vi "Get Plugin Name.vi"(8 "error in (no error)":errorcluster, 11 "Python Protocol in":refnum<class "Python Protocol.lvclass">) -> (0 "error out":errorcluster, 2 "String":string, 3 "Python Protocol out":refnum<class "Python Protocol.lvclass">)   [LabVIEW 2013, in "Python Protocol.lvlib" / "Python Protocol.lvclass"]
uses:
  Python Protocol.lvclass
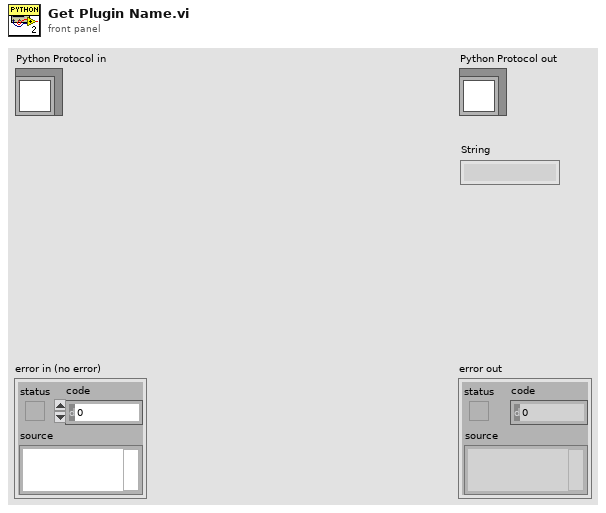
[diagram p1: front panel]
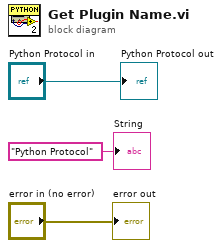
[diagram p0: block diagram]
diagram:
  "error out" <- "error in (no error)"
  "Python Protocol out" <- "Python Protocol in"
  "String" <- "Python Protocol" ("String")
